vi "MasterStateController.vi"() -> (3 "Confirmed States":bool[](array[boolean]), 4 "Disallowed States":bool[](array[boolean]), 5 "Master State Out":T1(ring)=enum."Trap")   [LabVIEW 2023]
doc: "This is the master robot state controller. The master robot state can affect any of the subsystem state controllers."
uses:
  3c4deeda-c82e-4bab-a34d-ad56dd11f424.vi
  GlobalDriverStationCommands.vi
  GlobalDriverStationData.vi
  GlobalElevator.vi
  GlobalNoteHandling.vi
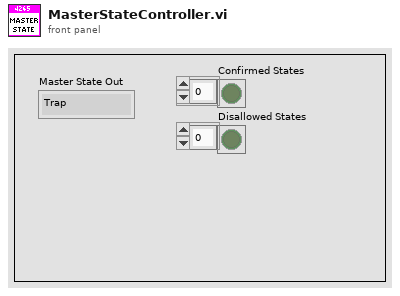
[diagram p1: front panel]
types:
  T1 = enum16{"Stow", "Speaker", "Amp", "Climbing", "Trap"}
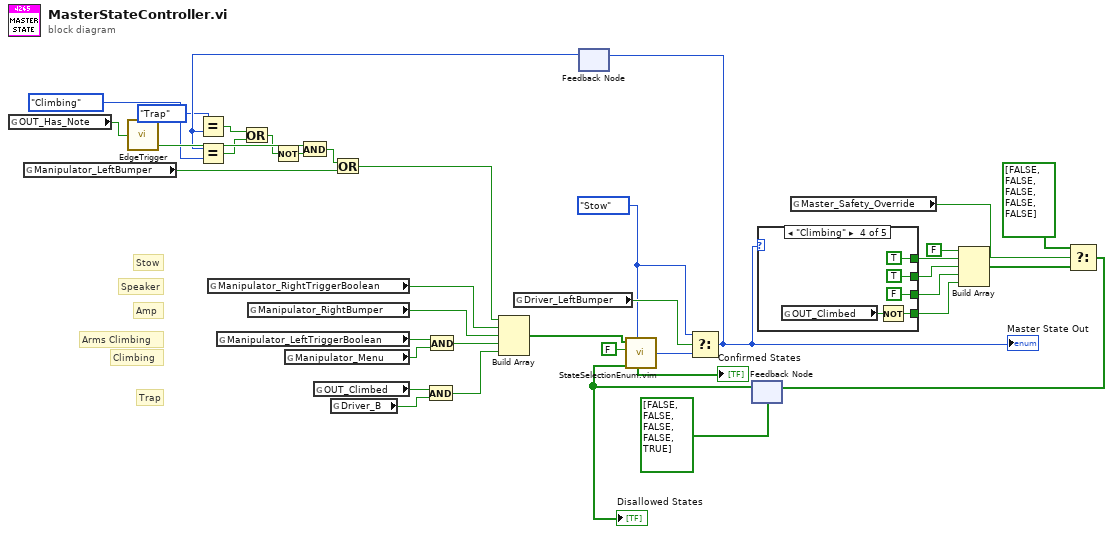
[diagram p0: block diagram]
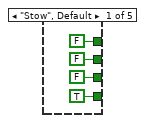
[diagram p2: hidden frame]
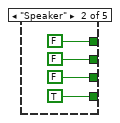
[diagram p3: hidden frame]
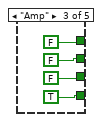
[diagram p4: hidden frame]
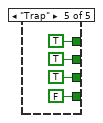
[diagram p5: hidden frame]
diagram:
  w18 = T1."Stow" ("Master State Out")
  # "Stow"
  # "Trap"
  # "Climbing"
  # "Arms Climbing"
  # "Amp"
  # "Speaker"
  n1 = global read "GlobalNoteHandling.vi" "OUT_Has_Note"() -> (w15:bool)
  n2 = global read "GlobalDriverStationCommands.vi" "Manipulator_LeftBumper"() -> (w16:bool)
  n3 = call "EdgeTrigger.vi"("Input Signal"=w15) -> ("Falling Edge Trigger"=w10:bool)  [unwired: 2 out]
  n4 = global read "GlobalDriverStationCommands.vi" "Manipulator_RightTriggerBoolean"() -> (w36:bool)
  n5 = global read "GlobalDriverStationCommands.vi" "Manipulator_LeftTriggerBoolean"() -> (w17:bool)
  n6 = global read "GlobalDriverStationCommands.vi" "Manipulator_RightBumper"() -> (w30:bool)
  n7 = global read "GlobalDriverStationCommands.vi" "Manipulator_Menu"() -> (w29:bool)
  n8 = global read "GlobalElevator.vi" "OUT_Climbed"() -> (w23:bool)
  n9 = global read "GlobalDriverStationCommands.vi" "Driver_B"() -> (w22:bool)
  n10 = And(x=w23, y=w22) -> (x .and. y?=w21:bool)
  n11 = And(x=w17, y=w29) -> (x .and. y?=w28:bool)
  n12 = global read "GlobalDriverStationCommands.vi" "Driver_LeftBumper"() -> (w19:bool)
  n13 = feedback #1() -> (w5:T1)  [unwired: 1 in]
  n14 = Equal?(x=T1."Trap", y=w5) -> (x = y?=w3:bool)
  n15 = Equal?(x=w5, y=T1."Climbing") -> (x = y?=w2:bool)
  n16 = Or(x=w3, y=w2) -> (x .or. y?=w1:bool)
  n17 = Not(x=w1) -> (.not. x?=w7:bool)
  n18 = And(x=w10, y=w7) -> (x .and. y?=w6:bool)
  n19 = Or(x=w6, y=w16) -> (x .or. y?=w14:bool)
  n20 = Build Array(w14, w36, w30, w28, w21) -> (w35:bool[])
  n21 = feedback #2(bool[] [FALSE, FALSE, FALSE, FALSE, TRUE]) -> (w12:bool[])
  "Disallowed States" <- w12
  n22 = call "StateSelectionEnum.vim"("Enum Def"=w18, "Disallowed States"=w12, "Enable Edge Trigger"=FALSE, "State Triggers"=w35) -> ("Selected State"=w38:T1, "Confirmed States"=→"Confirmed States":bool[])  [unwired: 1 in]
  n23 = Select(t=w18, s=w19, f=w38) -> (s? t:f=w9:T1)
  "Master State Out" <- w9
  n24 = feedback-in #1(w9) -> ()
  n25 = case shown="\"Climbing\"" w9 {
    tunnel: [TRUE ("OUT_Climbed") TRUE TRUE w51 FALSE ("OUT_Climbed")] -> w31
    tunnel: [FALSE FALSE FALSE FALSE TRUE] -> w32
    tunnel: [FALSE FALSE FALSE TRUE TRUE] -> w33
    tunnel: [FALSE FALSE FALSE TRUE TRUE] -> w34
    frame "Stow", Default {
    }
    frame "Speaker" {
    }
    frame "Amp" {
    }
    frame "Climbing" {
      n26 = global read "GlobalElevator.vi" "OUT_Climbed"() -> (w54:bool)
      n27 = Not(x=w54) -> (.not. x?=w51:bool)
    }
    frame "Trap" {
    }
  }
  n28 = global read "GlobalDriverStationData.vi" "Master_Safety_Override"() -> (w27:bool)
  n29 = Build Array(FALSE ("element"), w34, w33, w32, w31) -> (w25:bool[])
  n30 = Select(t=bool[] [FALSE, FALSE, FALSE, FALSE, FALSE], s=w27, f=w25) -> (s? t:f=w24:bool[])
  n31 = feedback-in #2(w24) -> ()
